vi "enum_moduleAdd.vi"(10 "in_modules":bool[](array[boolean]), 11 "enum_refin":refnum<vi>) -> (3 "enum_refout":refnum<vi>)   [LabVIEW 2014]
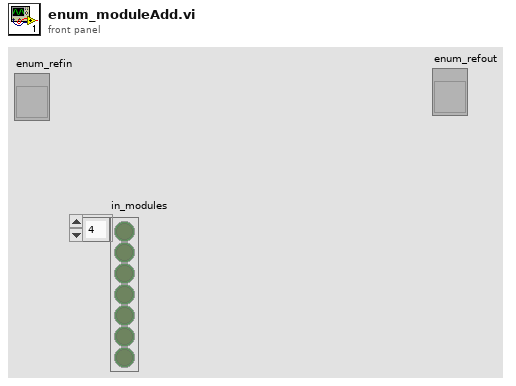
[diagram p1: front panel]
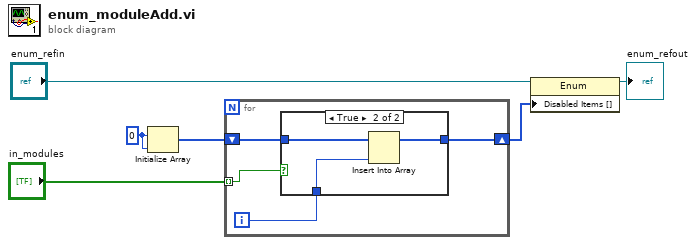
[diagram p0: block diagram]
diagram:
  w1 = 0 ("element")
  n1 = Initialize Array(w1, w1) -> (w5:i32[])
  n2 = for {
    tunnel: "in_modules" -> [w7] mode=indexing
    shift-right: [w9] -> w3
    shift-left: w5 -> [w10]
    i -> [w8]
    n3 = case shown="True" w7 {
      tunnel: w10 -> [w11 w14]
      tunnel: [w11 w13] -> w9
      tunnel: w8 -> [_ w12]
      frame False {
      }
      frame True {
        n4 = Insert Into Array(array=w14, new element=w12) -> (w13:i32[])  [unwired: 1 in]
      }
    }
  }
  n5 = property class="Enum"(reference="enum_refin", "Disabled Items []"=w3) -> (reference out=→"enum_refout":refnum<vi>)  [unwired: 1 in, 1 out]
